vi "LVRT Serial Close.vi"(8 "error out":errorcluster, 11 "FPGA Main Ref":T1) -> (0 "error out":errorcluster)   [LabVIEW 2009]
uses:
  serial FPGA main reference type def.ctl
  <vilib>/rvi/interface/nirviReadWriteControl/nirviReadWriteControl.xnode
  FPGA Bitfiles/Athena Brain.lvproj_FPGA Target 2_serial FPGA Main.vi.lvbitx
  serial FPGA Main.vi
  <vilib>/Utility/error.llb/Error Cluster From Error Code.vi
  <vilib>/rvi/errors/niLvFpgaAdjustHostInterfaceError.vi
  <vilib>/rvi/interface/common/niFpgaNodeNameForErrorReporting.ctl
  <vilib>/rvi/errors/niLvFpgaWhatHappensToTopLevelVI.ctl
  <vilib>/rvi/interface/nirviCloseFPGA/nirviCloseFPGA.xnode
  <vilib>/FPGAPlugInAG/sbRIO-9642/nirviIntfClose_sbRIO-9642.vi
  NiRioSrv.dll
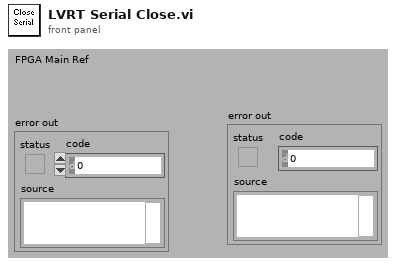
[diagram p1: front panel]
types:
  T1 = typedef "serial FPGA main reference type def.ctl" = refnum<k20>
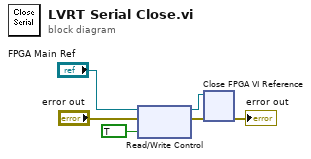
[diagram p0: block diagram]
diagram:
  n1 = xnode "Read/Write Control"("FPGA VI Reference In"="FPGA Main Ref", "error in"="error out", "stop"=TRUE) -> ("FPGA VI Reference Out"=w4:T1, "error out"=w5:errorcluster)
  n2 = xnode "Close FPGA VI Reference"("FPGA VI Reference In"=w4, "error in"=w5) -> ("error out"=→"error out":errorcluster)
